vi "Main.vi"() -> ()   [LabVIEW 2017]
doc: "This template is for the Queued Message Handler design pattern.\n\nThe Event Handling Loop generates messages based on user interface actions.\n\nThe Message Handling Loop processes messages generated by the Event Handling Loop, or by other messages. The messages are string values, so new messages can be added easily to the Message Cases case structure in the Message Handling Loop. Each message cluster can also provide an optional value for Message Data, which is a variant that can be converted to whatever message-specific data is required."
uses:
  controls/UI Data.ctl
  support/Message Queue/Enqueue Message (Single).vi
  <vilib>/MakerHub/LINX/Public/Utilities/Open Serial.vi
  <vilib>/Utility/error.llb/Error Cluster From Error Code.vi
  <vilib>/ErrorRing/Error Ring.xnode
  support/Message Queue/Message Queue.lvlib
  support/User Event - Stop/User Event - Stop.lvlib
  <vilib>/MakerHub/LINX/LMH-LINX.lvlib
panel:
  in  "Frequency (Hz)":dbl
  in  "DC/AC":bool
  in  "On-time (ms)":dbl
  in  "Start Button":bool
  in  "COM Port":refnum<visa-resource-name>="COM3"
  out "User Prompts":string="Initializing...."
  in  "Restart Button":bool
  in  "Exit":bool
  in  "Electrode Control":bool[][](array[boolean])=[[FALSE, FALSE, FALSE], [FALSE, FALSE, FALSE]]
  out "Error Out":errorcluster
  # "Digital Microfluidics HV Switching Control"
  # "Timing Controls"
  # "DC"
  # "AC"
  # "Program Status"
  # "Electrode Controls"
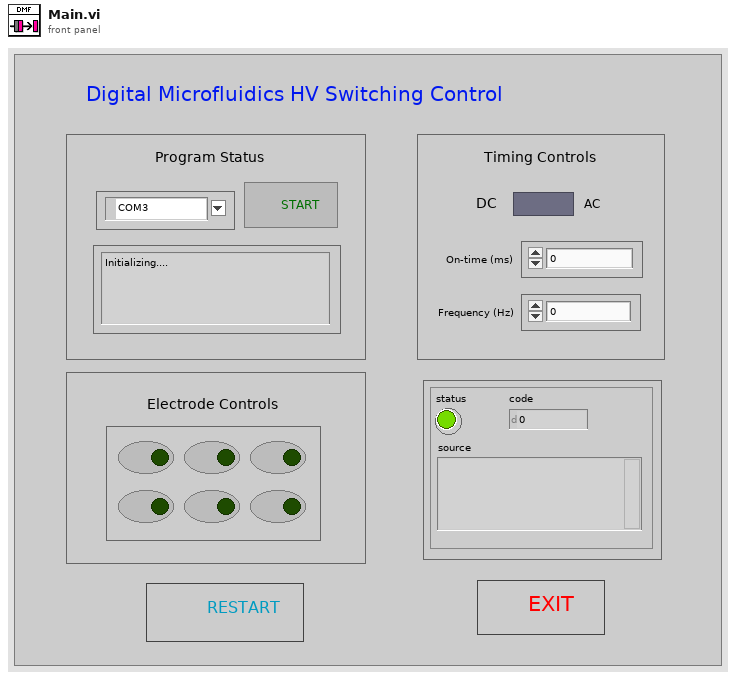
[diagram p1: front panel]
types:
  T1 = typedef "UI Data.ctl" = cluster{"VISA resource name":refnum<vi>, "Start Button":refnum<vi>, "DC/AC":refnum<vi>, "On-time (ms)":refnum<vi>, "Frequency (Hz)":refnum<vi>, "User Prompts":refnum<vi>, "Electrode Control":refnum<vi>, "Restart Button":refnum<vi>, "Exit":refnum<vi>}
  T2 = typedef "Message Queue.lvlib/All Message Queues.ctl" = cluster{"UI":refnum<queue>}
  T3 = typedef "LMH-LINX.lvlib/LINX Ref.ctl" = cluster{"IO":T4, "Interface":T5, "LINX Device Config":T6}
  T4 = typedef "LMH-LINX.lvlib/Platform.ctl" = enum16{"Remote", "Local"}
  T5 = typedef "LMH-LINX.lvlib/Interface.ctl" = enum16{"Serial", "TCP"}
  T6 = typedef "LMH-LINX.lvlib/Device.lvlib/LINX Device Config.ctl" = cluster{"Interface":T5, "COM Port":refnum<visa-resource-name>, "TCP Configuration":T7, "Device Family":u8, "Device ID":u8, "Device Name":string, "TCP Ref":refnum<k5>, "Channels":T8}
  T7 = typedef "LMH-LINX.lvlib/Device.lvlib/TCP Config.ctl" = cluster{"IP Address":string, "Port":u16}
  T8 = typedef "LMH-LINX.lvlib/Channels.ctl" = cluster{"DI":u8[], "DO":u8[], "AI":u8[], "AO":u8[], "PWM":u8[], "QE":u8[], "UART":u8[], "I2C 2":u8[], "SPI":u8[], "CAN":u8[], "Servo":u8[], "AI Ref (V)":dbl, "AI Resolution (Bits)":u8, "AO Ref (V)":dbl, "AO Resolution (Bits)":u8}
  T9 = cluster{i32, "index of element":i32, "Boolean":bool}
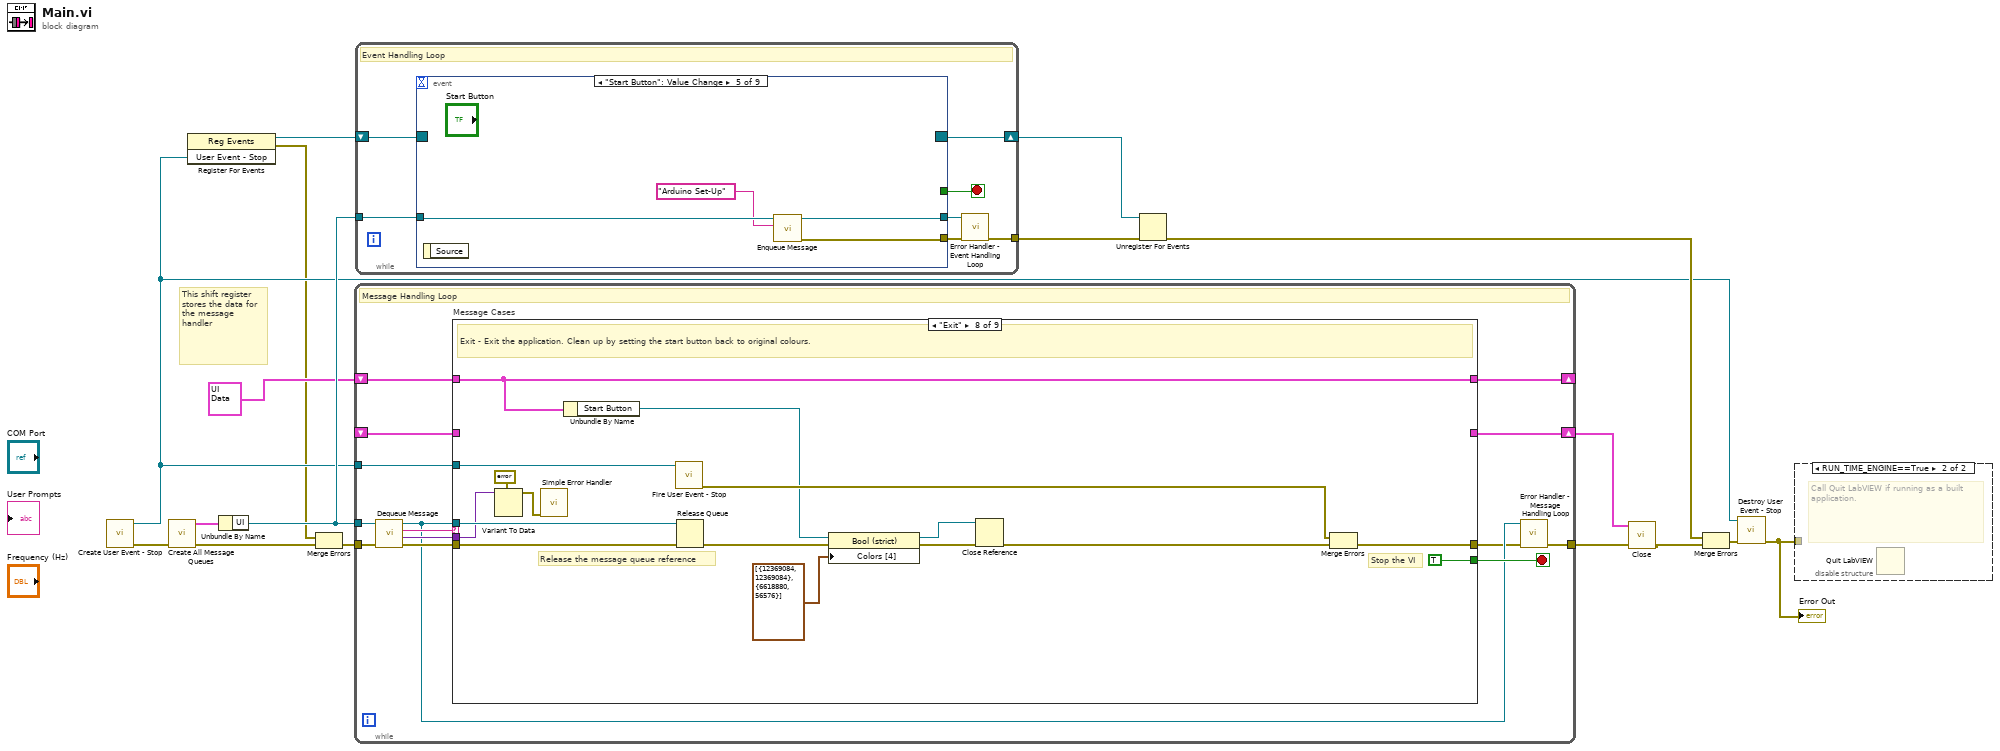
[diagram p0: block diagram]
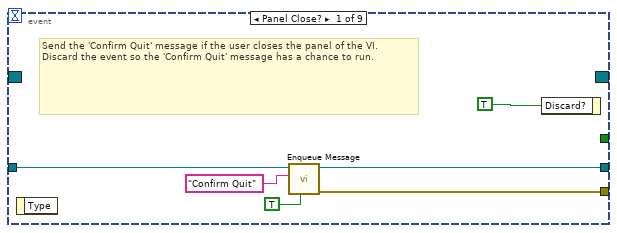
[diagram p3: hidden frame]
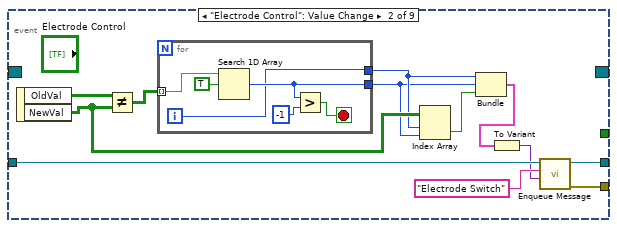
[diagram p4: hidden frame]
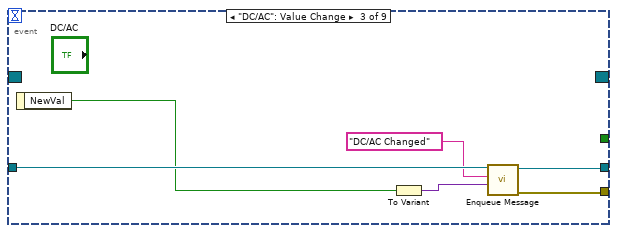
[diagram p5: hidden frame]
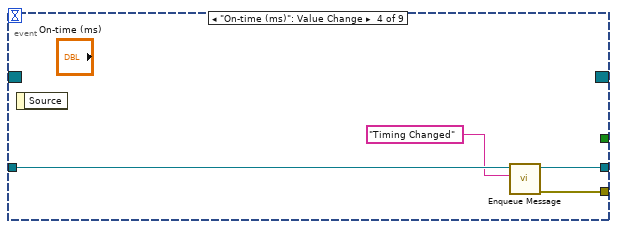
[diagram p6: hidden frame]
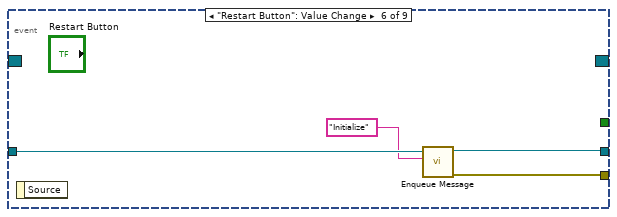
[diagram p7: hidden frame]
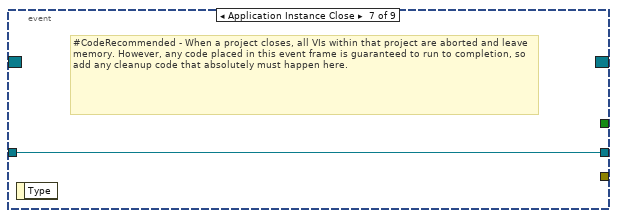
[diagram p8: hidden frame]
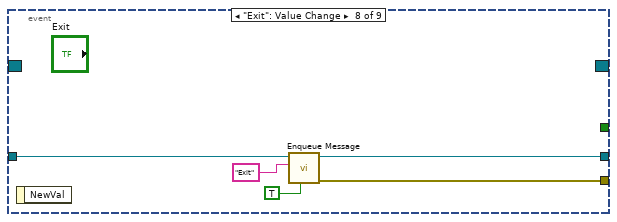
[diagram p9: hidden frame]
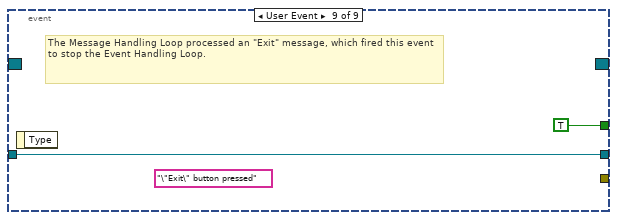
[diagram p10: hidden frame]
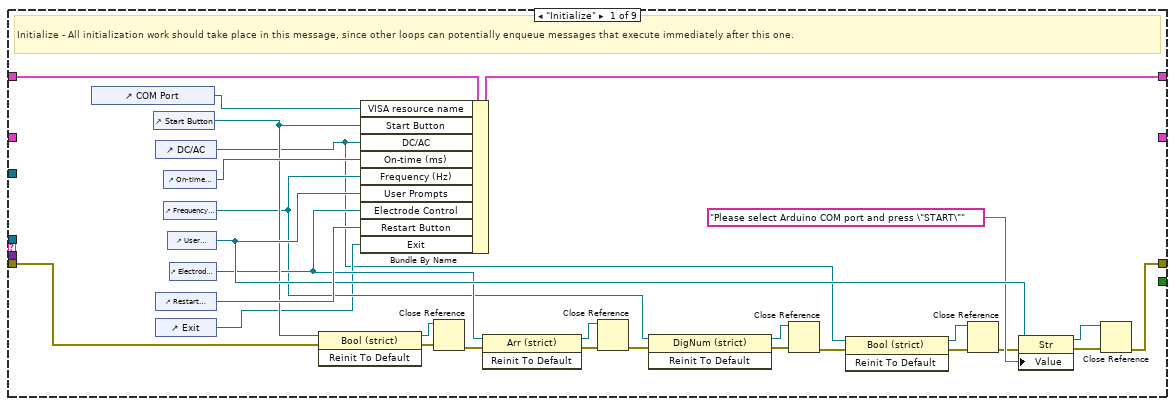
[diagram p11: hidden frame]
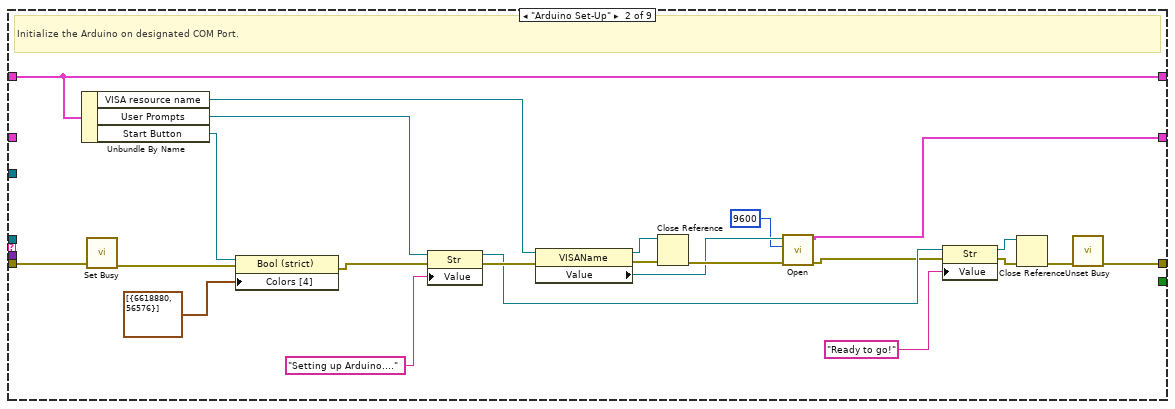
[diagram p12: hidden frame]
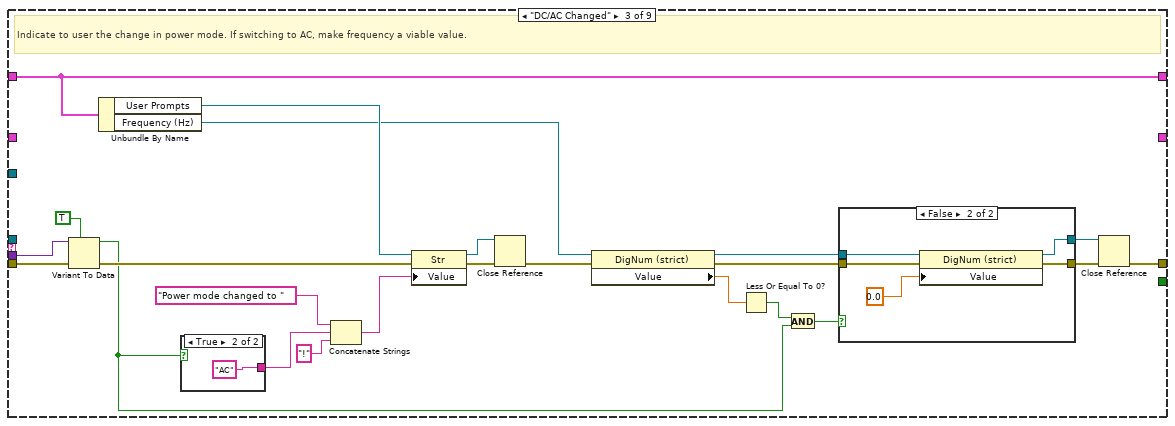
[diagram p13: hidden frame]
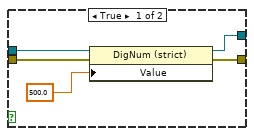
[diagram p14: hidden frame]
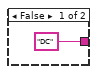
[diagram p15: hidden frame]
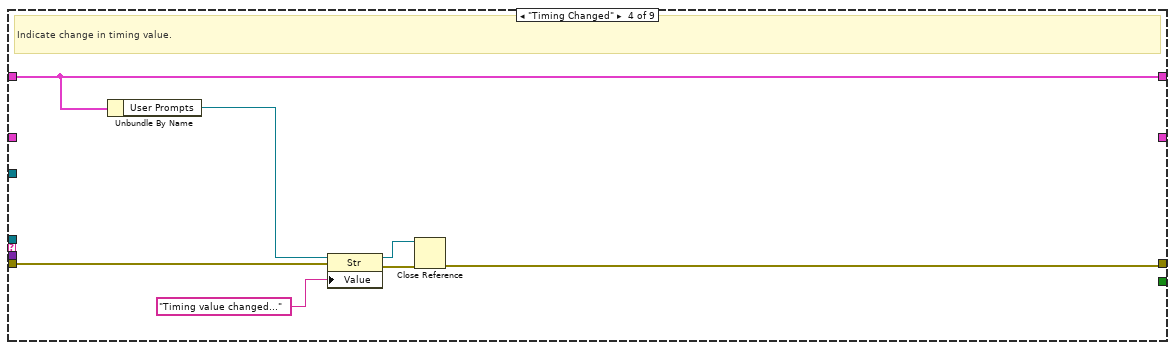
[diagram p16: hidden frame]
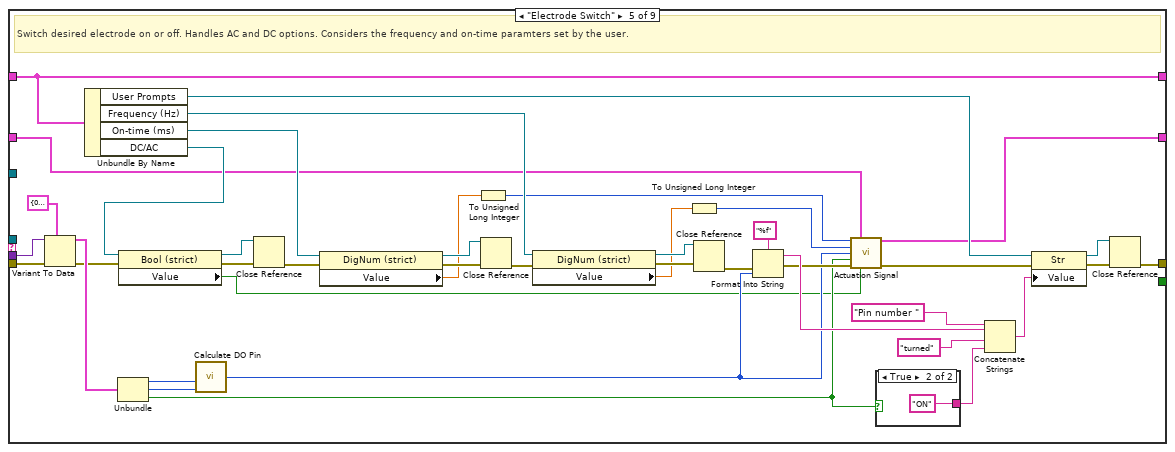
[diagram p17: hidden frame]
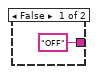
[diagram p18: hidden frame]
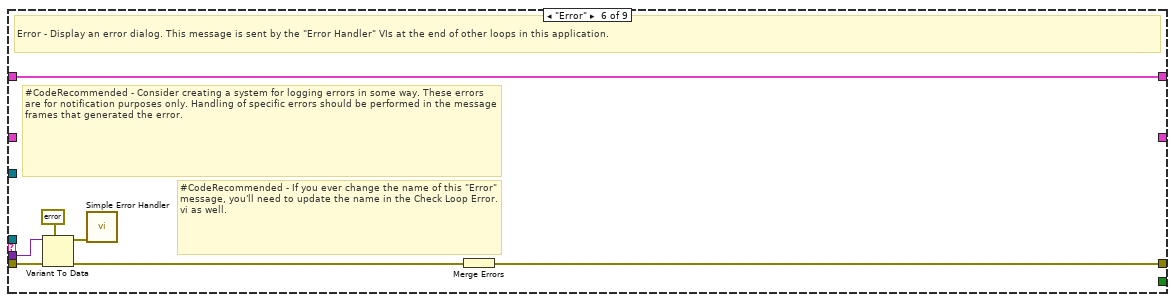
[diagram p19: hidden frame]
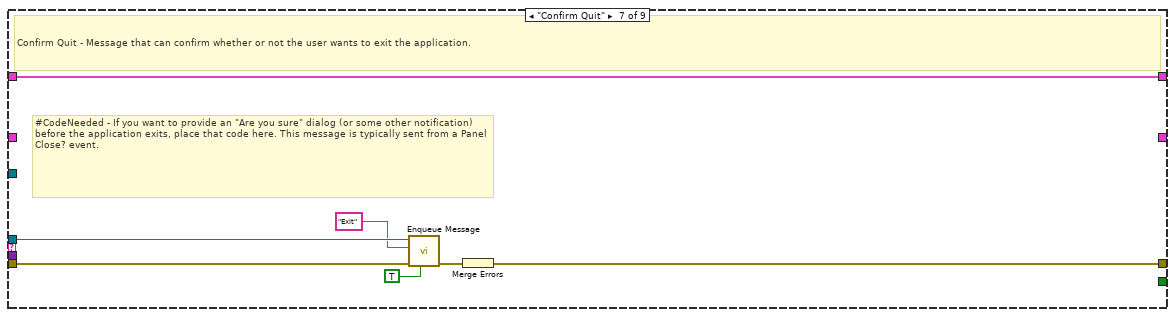
[diagram p20: hidden frame]
diagram:
  # "This shift register stores the data for the message handler"
  n1 = call "Create User Event - Stop.vi"() -> ("error out"=w14:errorcluster, "User Event - Stop"=w7:refnum<user-event>)  [unwired: 10 in]
  n2 = call "Create All Message Queues.vi"("error in (no error)"=w14) -> ("error out"=w17:errorcluster, "Message Queues out"=w16:T2)  [unwired: 9 in]
  n3 = register-events(w7) -> (reference out=w8:refnum<event-registration>, error out=w5:errorcluster)  [unwired: 2 in]
  n4 = Unbundle By Name(w16) -> ("UI"=w15:refnum<queue>)
  n5 = Merge Errors(w5, w17) -> (w6:errorcluster)
  n6 = while {
    tunnel: w15 -> [w23]
    shift-right: [w30] -> _
    shift-left: T1 {"VISA resource name"=refnum, "Start Button"=refnum, "DC/AC"=refnum, "On-time (ms)"=refnum, "Frequency (Hz)"=refnum, "User Prompts"=refnum, "Electrode Control"=refnum, "Restart Button"=refnum, "Exit"=refnum} ("Data Cluster") -> [w31]
    tunnel: w7 -> [w28]
    tunnel: w6 -> [w27]
    tunnel: [w21] -> w3
    shift-right: [w19] -> w1
    shift-left: _ -> [w18]
    stop <- w29 stop-if-true
    # "Message Handling Loop"
    n7 = call "Dequeue Message.vi"("error in (no error)"=w27, "Message Queue"=w23) -> ("error out"=w26:errorcluster, "Message Data"=w24:variant, "Message"=w25:string, "dup Message Queue"=w22:refnum<queue>)  [unwired: 6 in]
    n8 = case "Message Cases" shown="\"Exit\"" w25 {
      selector: w25 -> [_ _ _ _ _ _ _ _ w198]
      tunnel: w22 -> [_ _ _ _ _ _ w177 w197 _]
      tunnel: w26 -> [w49 w73 w104 w123 w165 w174 w181 w192 _]
      tunnel: [w50 w71 w84 w119 w155 w168 w179 w195 w199] -> w20
      tunnel: w31 -> [w59 w82 w105 w124 w159 w173 w180 w188 w200]
      tunnel: [w58 w82 w105 w124 w159 w173 w180 w188 w200] -> w30
      tunnel: [_ _ _ _ _ _ _ TRUE _] -> w29
      tunnel: w24 -> [_ _ w103 _ w164 w172 _ w189 _]
      tunnel: w28 -> [_ _ _ _ _ _ _ w194 _]
      tunnel: [_ w66 _ _ w126 _ _ _ _] -> w19
      tunnel: w18 -> [_ _ _ _ w125 _ _ _ _]
      frame "Initialize" {
        # "Initialize - All initialization work should take place in this message, since other loops can potentially enqueue messages that execute immediately after this one."
        n9 = control-ref of="COM Port"() -> (w56:refnum<vi>)
        n10 = control-ref of="Start Button"() -> (w48:refnum<vi>)
        n11 = control-ref of="DC/AC"() -> (w35:refnum<vi>)
        n12 = control-ref of="Restart Button"() -> (w55:refnum<vi>)
        n13 = control-ref of="Exit"() -> (w37:refnum<vi>)
        n14 = control-ref of="On-time (ms)"() -> (w57:refnum<vi>)
        n15 = control-ref of="Frequency (Hz)"() -> (w40:refnum<vi>)
        n16 = control-ref of="User Prompts"() -> (w54:refnum<vi>)
        n17 = control-ref of="Electrode Control"() -> (w45:refnum<vi>)
        n18 = invoke class="Bool (strict)" method="Reinit To Default"(reference=w48, error in=w49) -> (reference out=w46:refnum<vi>, error out=w47:errorcluster)  [unwired: 1 in, 1 out]
        n19 = Bundle By Name(cluster=w59, "VISA resource name"=w56, "Start Button"=w48, "DC/AC"=w35, "On-time (ms)"=w57, "Frequency (Hz)"=w40, "User Prompts"=w54, "Electrode Control"=w45, "Restart Button"=w55, "Exit"=w37) -> (w58:T1)
        n20 = Close Reference(reference=w46, error in (no error)=w47) -> (error out=w44:errorcluster)
        n21 = invoke class="Arr (strict)" method="Reinit To Default"(reference=w45, error in=w44) -> (reference out=w42:refnum<vi>, error out=w43:errorcluster)  [unwired: 1 in, 1 out]
        n22 = Close Reference(reference=w42, error in (no error)=w43) -> (error out=w41:errorcluster)
        n23 = invoke class="DigNum (strict)" method="Reinit To Default"(reference=w40, error in=w41) -> (reference out=w38:refnum<vi>, error out=w39:errorcluster)  [unwired: 1 in, 1 out]
        n24 = Close Reference(reference=w38, error in (no error)=w39) -> (error out=w36:errorcluster)
        n25 = invoke class="Bool (strict)" method="Reinit To Default"(reference=w35, error in=w36) -> (reference out=w32:refnum<vi>, error out=w34:errorcluster)  [unwired: 1 in, 1 out]
        n26 = Close Reference(reference=w32, error in (no error)=w34) -> (error out=w33:errorcluster)
        n27 = property class="Str"(reference=w54, error in=w33, "Value"="Please select Arduino COM port and press \"START\"") -> (reference out=w52:refnum<vi>, error out=w53:errorcluster)
        n28 = Close Reference(reference=w52, error in (no error)=w53) -> (error out=w50:errorcluster)
      }
      frame "Arduino Set-Up" {
        # "Initialize the Arduino on designated COM Port."
        n29 = Unbundle By Name(w82) -> ("VISA resource name"=w81:refnum<vi>, "User Prompts"=w75:refnum<vi>, "Start Button"=w62:refnum<vi>)
        n30 = call <vilib>:"Set Busy.vi"("error in (no error)"=w73) -> ("error out"=w63:errorcluster)  [unwired: 9 in, 1 out]
        n31 = property class="Bool (strict)"(reference=w62, error in=w63, "Colors [4]"=cluster{u32, u32}[] [{6618880, 56576}]) -> (error out=w61:errorcluster)  [unwired: 1 out]
        n32 = property class="Str"(reference=w75, error in=w61, "Value"="Setting up Arduino....") -> (reference out=w69:refnum<vi>, error out=w70:errorcluster)
        n33 = property class="VISAName"(reference=w81, error in=w70) -> (reference out=w79:refnum<vi>, error out=w80:errorcluster, "Value"=w67:refnum<visa-resource-name>)
        n34 = Close Reference(reference=w79, error in (no error)=w80) -> (error out=w68:errorcluster)
        n35 = call-poly <vilib>:"Open.vi"("Error In"=w68, "Baud Rate Override"=u32 9600, "Serial Port"=w67) -> ("Error Out"=w65:errorcluster, "LINX Resource"=w66:T3)  [unwired: 6 in, 1 out]
        n36 = property class="Str"(reference=w69, error in=w65, "Value"="Ready to go!") -> (reference out=w77:refnum<vi>, error out=w78:errorcluster)
        n37 = Close Reference(reference=w77, error in (no error)=w78) -> (error out=w72:errorcluster)
        n38 = call <vilib>:"Unset Busy.vi"("error in (no error)"=w72) -> ("error out"=w71:errorcluster)  [unwired: 10 in]
      }
      frame "DC/AC Changed" {
        # "Indicate to user the change in power mode. If switching to AC, make frequency a viable value."
        n39 = Variant To Data(error in=w104, type=TRUE, Variant=w103) -> (data=w89:bool, error out=w99:errorcluster)
        n40 = Unbundle By Name(w105) -> ("User Prompts"=w96:refnum<vi>, "Frequency (Hz)"=w92:refnum<vi>)
        n41 = case shown="True" w89 {
          tunnel: ["DC" "AC"] -> w100
          frame False {
          }
          frame True {
          }
        }
        n42 = Concatenate Strings("Power mode changed to " ("string"), w100, "!") -> (w95:string)
        n43 = property class="Str"(reference=w96, error in=w99, "Value"=w95) -> (reference out=w97:refnum<vi>, error out=w98:errorcluster)
        n44 = Close Reference(reference=w97, error in (no error)=w98) -> (error out=w93:errorcluster)
        n45 = property class="DigNum (strict)"(reference=w92, error in=w93) -> (reference out=w86:refnum<vi>, error out=w87:errorcluster, "Value"=w91:dbl)
        n46 = Less Or Equal To 0?(x=w91) -> (x <= 0?=w90:bool)
        n47 = And(x=w90, y=w89) -> (x .and. y?=w88:bool)
        n48 = case shown="False" w88 {
          tunnel: w87 -> [w110 w115]
          tunnel: w86 -> [w109 w114]
          tunnel: [w107 w112] -> w85
          tunnel: [w106 w111] -> w83
          frame True {
            n49 = property class="DigNum (strict)"(reference=w109, error in=w110, "Value"=500.0) -> (reference out=w106:refnum<vi>, error out=w107:errorcluster)
          }
          frame False {
            n50 = property class="DigNum (strict)"(reference=w114, error in=w115, "Value"=0.0) -> (reference out=w111:refnum<vi>, error out=w112:errorcluster)
          }
        }
        n51 = Close Reference(reference=w83, error in (no error)=w85) -> (error out=w84:errorcluster)
      }
      frame "Timing Changed" {
        # "Indicate change in timing value."
        n52 = Unbundle By Name(w124) -> ("User Prompts"=w122:refnum<vi>)
        n53 = property class="Str"(reference=w122, error in=w123, "Value"="Timing value changed...") -> (reference out=w120:refnum<vi>, error out=w121:errorcluster)
        n54 = Close Reference(reference=w120, error in (no error)=w121) -> (error out=w119:errorcluster)
      }
      frame "Electrode Switch" {
        # "Switch desired electrode on or off. Handles AC and DC options. Considers the frequency and on-time paramters set by the user."
        n55 = Variant To Data(error in=w165, type=cluster{i32, i32, bool} {0, 0, FALSE}, Variant=w164) -> (data=w162:cluster{i32, i32, bool}, error out=w154:errorcluster)
        n56 = Unbundle By Name(w159) -> ("User Prompts"=w156:refnum<vi>, "Frequency (Hz)"=w135:refnum<vi>, "On-time (ms)"=w136:refnum<vi>, "DC/AC"=w137:refnum<vi>)
        n57 = Unbundle(w162) -> (w161:i32, w160:i32, w128:bool)
        n58 = property class="Bool (strict)"(reference=w137, error in=w154) -> (reference out=w152:refnum<vi>, error out=w153:errorcluster, "Value"=w127:bool)
        n59 = call "Calculate DO Pin.vi"("Row"=w161, "Col"=w160) -> ("MC Pin"=w133:u8)  [unwired: 3 in]
        n60 = Close Reference(reference=w152, error in (no error)=w153) -> (error out=w151:errorcluster)
        n61 = property class="DigNum (strict)"(reference=w136, error in=w151) -> (reference out=w149:refnum<vi>, error out=w150:errorcluster, "Value"=w142:dbl)
        n62 = To Unsigned Long Integer(number=w142) -> (unsigned 32bit integer=w130:u32)
        n63 = Close Reference(reference=w149, error in (no error)=w150) -> (error out=w134:errorcluster)
        n64 = property class="DigNum (strict)"(reference=w135, error in=w134) -> (reference out=w139:refnum<vi>, error out=w140:errorcluster, "Value"=w132:dbl)
        n65 = To Unsigned Long Integer(number=w132) -> (unsigned 32bit integer=w131:u32)
        n66 = Close Reference(reference=w139, error in (no error)=w140) -> (error out=w138:errorcluster)
        n67 = Format Into String(format string="%f", error in=w138, w133) -> (resulting string=w146:string, error out=w141:errorcluster)  [unwired: 1 in]
        n68 = call "Actuation Signal.vi"("On-time (ms)"=w130, "LINX Resource"=w125, "Frequency"=w131, "Pin Number"=w133, "On or Off?"=w128, "Error In"=w141, "DC or AC?"=w127) -> ("LINX Resource Out"=w126:T3, "Error Out"=w129:errorcluster)  [unwired: 7 in]
        n69 = case shown="True" w128 {
          tunnel: ["OFF" "ON"] -> w144
          frame False {
          }
          frame True {
          }
        }
        n70 = Concatenate Strings("Pin number " ("string"), w146, "turned" ("string"), w144) -> (w143:string)
        n71 = property class="Str"(reference=w156, error in=w129, "Value"=w143) -> (reference out=w157:refnum<vi>, error out=w158:errorcluster)
        n72 = Close Reference(reference=w157, error in (no error)=w158) -> (error out=w155:errorcluster)
      }
      frame "Error" {
        # "#CodeRecommended - If you ever change the name of this \"Error\" message, you'll need to update the name in the Check Loop Error.vi as well."
        # "#CodeRecommended - Consider creating a system for logging errors in some way. These errors are for notification purposes only. Handling of specific errors should be performed in the message frames that generated the error."
        # "Error - Display an error dialog. This message is sent by the \"Error Handler\" VIs at the end of other loops in this application."
        n73 = Variant To Data(error in=w174, type=errorcluster {"status"=FALSE, "code"=0, "source"=""} ("error constant"), Variant=w172) -> (data=w170:errorcluster, error out=w169:errorcluster)
        n74 = call <vilib>:"Simple Error Handler.vi"("error in (no error)"=w170) -> ()  [unwired: 4 in, 5 out]
        n75 = Merge Errors(w169) -> (w168:errorcluster)
      }
      frame "Confirm Quit" {
        # "#CodeNeeded - If you want to provide an \"Are you sure\" dialog (or some other notification) before the application exits, place that code here. This message is typically sent from a Panel Close? event."
        # "Confirm Quit - Message that can confirm whether or not the user wants to exit the application."
        n76 = call-poly "Enqueue Message.vi"("Priority Message? (F)"=TRUE, "error in (no error)"=w181, "Message"="Exit", "Message Queue"=w177) -> ("error out"=w178:errorcluster)  [unwired: 6 in, 1 out]
        n77 = Merge Errors(w178) -> (w179:errorcluster)
      }
      frame "Exit" {
        # "Stop the VI"
        # "Release the message queue reference"
        # "Exit - Exit the application. Clean up by setting the start button back to original colours."
        n78 = Variant To Data(type=errorcluster {"status"=FALSE, "code"=0, "source"=""} ("error constant"), Variant=w189) -> (data=w190:errorcluster)  [unwired: 1 in, 1 out]
        n79 = call <vilib>:"Simple Error Handler.vi"("error in (no error)"=w190) -> ()  [unwired: 4 in, 5 out]
        n80 = Unbundle By Name(w188) -> ("Start Button"=w186:refnum<vi>)
        n81 = call "Fire User Event - Stop.vi"("User Event - Stop"=w194) -> ("error out"=w193:errorcluster)  [unwired: 10 in]
        n82 = Release Queue(queue=w197, error in (no error)=w192) -> (error out=w187:errorcluster)  [unwired: 1 in, 2 out]
        n83 = property class="Bool (strict)"(reference=w186, error in=w187, "Colors [4]"=cluster{u32, u32}[] [{12369084, 12369084}, {6618880, 56576}]) -> (reference out=w184:refnum<vi>, error out=w185:errorcluster)
        n84 = Close Reference(reference=w184, error in (no error)=w185) -> (error out=w183:errorcluster)
        n85 = Merge Errors(w193, w183) -> (w195:errorcluster)
      }
      frame Default {
        # "'Default' case only runs if there is a message that isn't defined in any of the other cases.  Output a programming error."
        n86 = xnode "Error Ring"("parameter 0"=w198) -> ("error out"=w199:errorcluster)
      }
    }
    n87 = call "Error Handler - Message Handling Loop.vi"("error in (no error)"=w20, "Message Queue"=w22) -> ("dup error in"=w21:errorcluster)  [unwired: 8 in, 1 out]
  }
  n88 = while {
    tunnel: w15 -> [w214]
    shift-right: [w212] -> w11
    shift-left: w8 -> [w213]
    tunnel: [w208] -> w9
    stop <- w210 stop-if-true
    # "Event Handling Loop"
    n89 = event shown="[4] \"Start Button\": Value Change" {
      selector: w213 -> [_ _ _ _ _ _ _ _ _]
      dyn-events: [_ _ _ _ _ _ _ _ _] -> w212
      timeout: _ -> [_ _ _ _ _ _ _ _ _]
      tunnel: [_ _ _ _ _ _ _ _ TRUE ("Discard?")] -> w210
      tunnel: w214 -> [w219 w232 w243 w246 w251 w256 w257 w262 w264]
      tunnel: [w218 w230 w244 w247 w250 w254 _ w261 _] -> w211
      tunnel: [w217 w231 w242 w248 w252 w255 w257 w260 w264] -> w209
      event Panel Close? {
        # "Send the 'Confirm Quit' message if the user closes the panel of the VI. Discard the event so the 'Confirm Quit' message has a chance to run."
        n90 = event-data() -> ()  [unwired: 1 in, 1 out]
        n91 = call-poly "Enqueue Message.vi"("Priority Message? (F)"=TRUE, "Message"="Confirm Quit", "Message Queue"=w219) -> ("error out"=w218:errorcluster, "dup Message Queue"=w217:refnum<queue>)  [unwired: 7 in]
        n92 = event-data("Discard?"=TRUE) -> ()  [unwired: 1 in, 1 out]
      }
      event "Electrode Control": Value Change {
        n93 = event-data() -> ("OldVal"=w229:bool[][], "NewVal"=w226:bool[][])  [unwired: 1 in]
        n94 = Not Equal?(x=w229, y=w226) -> (x != y?=w228:bool[][])
        n95 = for {
          tunnel: w228 -> [w238] mode=indexing
          tunnel: [w236] -> w224
          tunnel: [w233] -> w225
          i -> [w233]
          stop <- w234 stop-if-true
          n96 = Search 1D Array(1D array=w238, element=TRUE) -> (index of element=w236:i32)  [unwired: 1 in]
          n97 = Greater?(x=w236, y=-1) -> (0:w234:bool)
        }
        n98 = Index Array(array=w226, index (row)=w225, index (col)=w224) -> (element=w223:bool)
        n99 = Bundle(w225, "index of element"=w224, "Boolean"=w223) -> (w222:T9)  [unwired: 1 in]
        n100 = To Variant(anything=w222) -> (Variant=w221:variant)
        n101 = call-poly "Enqueue Message.vi"("Message Data"=w221, "Message"="Electrode Switch", "Message Queue"=w232) -> ("error out"=w230:errorcluster, "dup Message Queue"=w231:refnum<queue>)  [unwired: 7 in]
      }
      event "DC/AC": Value Change {
        n102 = event-data() -> ("NewVal"=w241:bool)  [unwired: 1 in]
        n103 = To Variant(anything=w241) -> (Variant=w240:variant)
        n104 = call-poly "Enqueue Message.vi"("Message Data"=w240, "Message"="DC/AC Changed", "Message Queue"=w243) -> ("error out"=w244:errorcluster, "dup Message Queue"=w242:refnum<queue>)  [unwired: 7 in]
      }
      event "On-time (ms)": Value Change {
        n105 = event-data() -> ()  [unwired: 1 in, 1 out]
        n106 = call-poly "Enqueue Message.vi"("Message"="Timing Changed", "Message Queue"=w246) -> ("error out"=w247:errorcluster, "dup Message Queue"=w248:refnum<queue>)  [unwired: 8 in]
      }
      event "Start Button": Value Change {
        n107 = event-data() -> ()  [unwired: 1 in, 1 out]
        n108 = call-poly "Enqueue Message.vi"("Message"="Arduino Set-Up", "Message Queue"=w251) -> ("error out"=w250:errorcluster, "dup Message Queue"=w252:refnum<queue>)  [unwired: 8 in]
      }
      event "Restart Button": Value Change {
        n109 = event-data() -> ()  [unwired: 1 in, 1 out]
        n110 = call-poly "Enqueue Message.vi"("Message"="Initialize", "Message Queue"=w256) -> ("error out"=w254:errorcluster, "dup Message Queue"=w255:refnum<queue>)  [unwired: 8 in]
      }
      event Application Instance Close {
        # "#CodeRecommended - When a project closes, all VIs within that project are aborted and leave memory. However, any code placed in this event frame is guaranteed to run to completion, so add any cleanup code that absolutely must happen here."
        n111 = event-data() -> ()  [unwired: 1 in, 1 out]
      }
      event "Exit": Value Change {
        n112 = event-data() -> ()  [unwired: 1 in, 1 out]
        n113 = call-poly "Enqueue Message.vi"("Priority Message? (F)"=TRUE, "Message"="Exit", "Message Queue"=w262) -> ("error out"=w261:errorcluster, "dup Message Queue"=w260:refnum<queue>)  [unwired: 7 in]
      }
      event User Event {
        (unwired) "\"Exit\" button pressed" ("VI Stopped")
        # "The Message Handling Loop processed an \"Exit\" message, which fired this event to stop the Event Handling Loop."
        n114 = event-data() -> ()  [unwired: 1 in, 1 out]
      }
    }
    n115 = call "Error Handler - Event Handling Loop.vi"("error in (no error)"=w211, "Message Queue"=w209) -> ("dup error in"=w208:errorcluster)  [unwired: 8 in, 1 out]
  }
  n116 = Unregister For Events(event registration refnum=w11, error in=w9) -> (error out=w12:errorcluster)
  n117 = call <vilib>:"Close.vi"("Error In"=w3, "LINX Resource"=w1) -> ("Error Out"=w2:errorcluster)  [unwired: 9 in]
  n118 = Merge Errors(w12, w2) -> (w13:errorcluster)
  n119 = call "Destroy User Event - Stop.vi"("error in (no error)"=w13, "User Event - Stop"=w7) -> ("error out"=w4:errorcluster)  [unwired: 9 in]
  "Error Out" <- w4
  n120 = disable-structure shown="RUN_TIME_ENGINE==True" {
    disable-tunnel: w4 -> [_ _]
    frame condition #0 (active) {
    }
    frame condition #1 {
      # "Call Quit LabVIEW if running as a built application."
      n121 = Quit LabVIEW() -> ()  [unwired: 1 in]
    }
  }
